vi "Cache_Info Load.vi"(0 "Refnum in":T2, 5 "Class Name":string, 11 "error in (no error)":errorcluster) -> (4 "Refnum out":T2, 6 "Class Info":T1, 8 "Is Interface":bool, 10 "Success?":bool, 15 "error out":errorcluster)   [LabVIEW 2019, in "ClassLoader.lvlib"]
uses:
  ClassLoader.lvlib
  <vilib>/Utility/config.llb/NI_LVConfig.lvlib
  <vilib>/Utility/config.llb/Read Key (String).vi
  Ctl/Ctl_Class Info.ctl
  <vilib>/Utility/config.llb/Read Key (Boolean).vi
  <vilib>/Utility/config.llb/Config Data RefNum.ctl
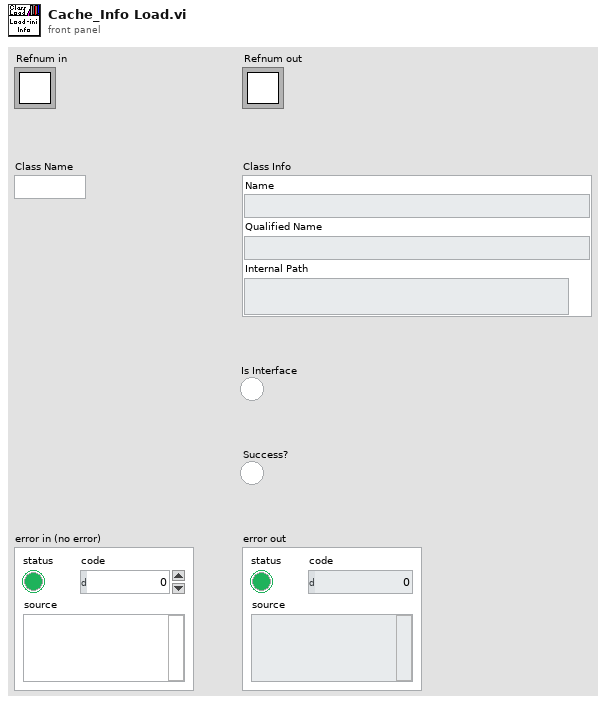
[diagram p1: front panel]
types:
  T1 = typedef "ClassLoader.lvlib/Ctl_Class Info.ctl" = cluster{"Name":string, "Qualified Name":string, "Internal Path":string}
  T2 = typedef "NI_LVConfig.lvlib/Config Data RefNum.ctl" = refnum<k1>
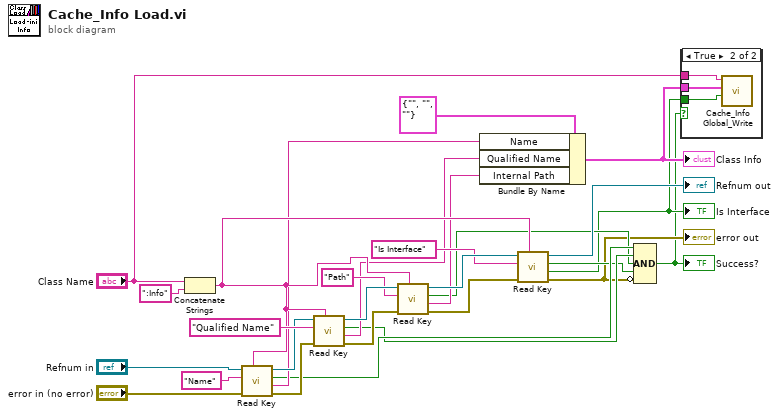
[diagram p0: block diagram]
diagram:
  n1 = Concatenate Strings("Class Name", ":Info" ("string")) -> (w17:string)
  n2 = call-poly <vilib>:"Read Key.vi"("section"=w17, "error in (no error)"="error in (no error)", "key"="Name", "refnum"="Refnum in") -> ("error out"=w26:errorcluster, "value"=w13:string, "found?"=w9:bool, "refnum out"=w24:T2)  [unwired: 4 in]
  n3 = call-poly <vilib>:"Read Key.vi"("section"=w17, "error in (no error)"=w26, "key"="Qualified Name", "refnum"=w24) -> ("error out"=w21:errorcluster, "value"=w12:string, "found?"=w8:bool, "refnum out"=w23:T2)  [unwired: 4 in]
  n4 = call-poly <vilib>:"Read Key.vi"("section"=w17, "error in (no error)"=w21, "key"="Path", "refnum"=w23) -> ("error out"=w18:errorcluster, "value"=w11:string, "found?"=w7:bool, "refnum out"=w20:T2)  [unwired: 4 in]
  n5 = Bundle By Name(cluster=T1 {"Name"="", "Qualified Name"="", "Internal Path"=""} ("Class Info"), "Name"=w13, "Qualified Name"=w12, "Internal Path"=w11) -> (w4:T1)
  "Class Info" <- w4
  n6 = call-poly <vilib>:"Read Key.vi"("section"=w17, "error in (no error)"=w18, "key"="Is Interface", "refnum"=w20) -> ("error out"=w5:errorcluster, "value"=w3:bool, "found?"=w6:bool, "refnum out"=→"Refnum out":T2)  [unwired: 4 in]
  "error out" <- w5
  "Is Interface" <- w3
  n7 = Compound Arithmetic op=AND(w9, w8, w7, w6, invert w5) -> (w2:bool)
  "Success?" <- w2
  n8 = case shown="True" w2 {
    tunnel: w4 -> [_ w31]
    tunnel: w3 -> [_ w30]
    tunnel: "Class Name" -> [_ w29]
    frame False {
    }
    frame True {
      n9 = call "Cache_Info Global_Write.vi"("Is Interface?"=w30, "Class Info"=w31, "Class Name"=w29) -> ()  [unwired: 9 in]
    }
  }
